vi "Host_HealthCheck_convertCluster.vi"(11 "Data":T1={"cRIO Data"={"HallEffect Right (cm)"=0.0, "HallEffect Left (cm)"=0.0, "Optical Sensor 1 (V)"=0.0, "Optical Sensor 2 (V)"=0.0, "24V Voltage  (V)"=0.0, "24V Current (A)"=0.0, "Contactor H1 Continuity"=0.0, "Contactor L1 Continuity "=0.0, "Contactor H2 Continuity"=0.0, "Contactor L2 Continuity "=0.0, "Brake PT(psig)"=0.0, "Pump PT (psig)"=0.0, "24V Temp   (C)"=0.0, "Tank PT(psig) "=0.0, "ABS Pressure 1 (psig)"=0.0, "ABS Pressure 2 (psig) "=0.0, "Displacement (ft)"=0.0, "Velocity (ft/s)"=0.0, "Time (ms)"=0.0, "PV 1 Temp"=0.0, "PV2 Temp"=0.0}, "IMU Data"={"y acceleration (g)"=0.0, "Pressure (psia)"=0.0, "Temperature (F)"=0.0}, "BMS Data"={"Pack 1 Max Cell\n Voltage (V)"=0.0, "Pack 1 Max Cell\n ID "=0.0, "Pack 1 Min Cell \nVoltage (V)"=0.0, "Pack 1 Min Cell \nID "=0.0, "Pack 1 State of Charge  (%)"=0.0, "Pack 1 Average Voltage1 (V)"=0.0, "Pack 1Voltage Delta (V)"=0.0, "Pack 1 Current (A)"=0.0, "Pack 1 Voltage (V)"=0.0, "Pack 1 Max Resistance (Ohm)"=0.0, "Pack 1Min Resistance (Ohm)"=0.0, "Pack 1Average Resistance (Ohm)"=0.0, "Pack 1Delta Resistance (Ohm)"=0.0, "Pack 1 Highest Temperature(F)"=0.0, "BmsStatus1"={"isFault"=FALSE, "isolationMonitoring"=FALSE}, "Pack 2 Max Cell\n Voltage (V) "=0.0, "Pack 2 Max Cell\n ID  "=0.0, "Pack 2 Min Cell \nVoltage (V) "=0.0, "Pack 2 Min Cell \nID  "=0.0, "Pack 2 Average Voltage1 (V)"=0.0, "Pack 2 Voltage Delta (V) "=0.0, "Pack 2 Current (A)"=0.0, "Pack 2 Voltage (V) "=0.0, "Pack 2 State of Charge  (%) "=0.0, "Pack 2 Max Resistance (Ohm) "=0.0, "Pack 2 Min Resistance (Ohm)"=0.0, "Pack 2 Average Resistance (Ohm)"=0.0, "Pack 2 Delta Resistance (Ohm) "=0.0, "Pack 2 Highest Temperature(F) "=0.0, "BmsStatus 2"={"isFault"=FALSE, "isolationMonitoring"=FALSE}}, "Motor Data"={" Velocity (RPM)"=0.0, " MotorTemp(C)"=0.0, " ControlTemp(C)"=0.0, " DcLinkVolt(V)"=0.0, " ErrorCode"=0.0, "IsAlive"=FALSE, "motorStatus"={"isReady"=FALSE, "isOn"=FALSE, "isOperEn"=FALSE, "isFault"=FALSE, "isVoltEn"=FALSE, "targetReached"=FALSE, "isWarning"=FALSE}, "motorControllerState"=1}} {"Motor Data"."motorControllerState" items=["unknown"=1, "boot-up"=0, "stopped"=4, "operational"=5, "pre-operational"=127, "connection lost"=128]}) -> (3 "Array":dbl[](array[numeric]))   [LabVIEW 2018]
uses:
  Type_Def/TypeDef_cRIODatas.ctl
  Type_Def/TypeDef_BMSDatas.ctl
  Type_Def/Master_DataControl.ctl
  Type_Def/TypeDef FixedMotorData.ctl
  Type_Def/Type_Def IMUDatas.ctl
  Type_Def/TypeDef_BMSStatuss.ctl
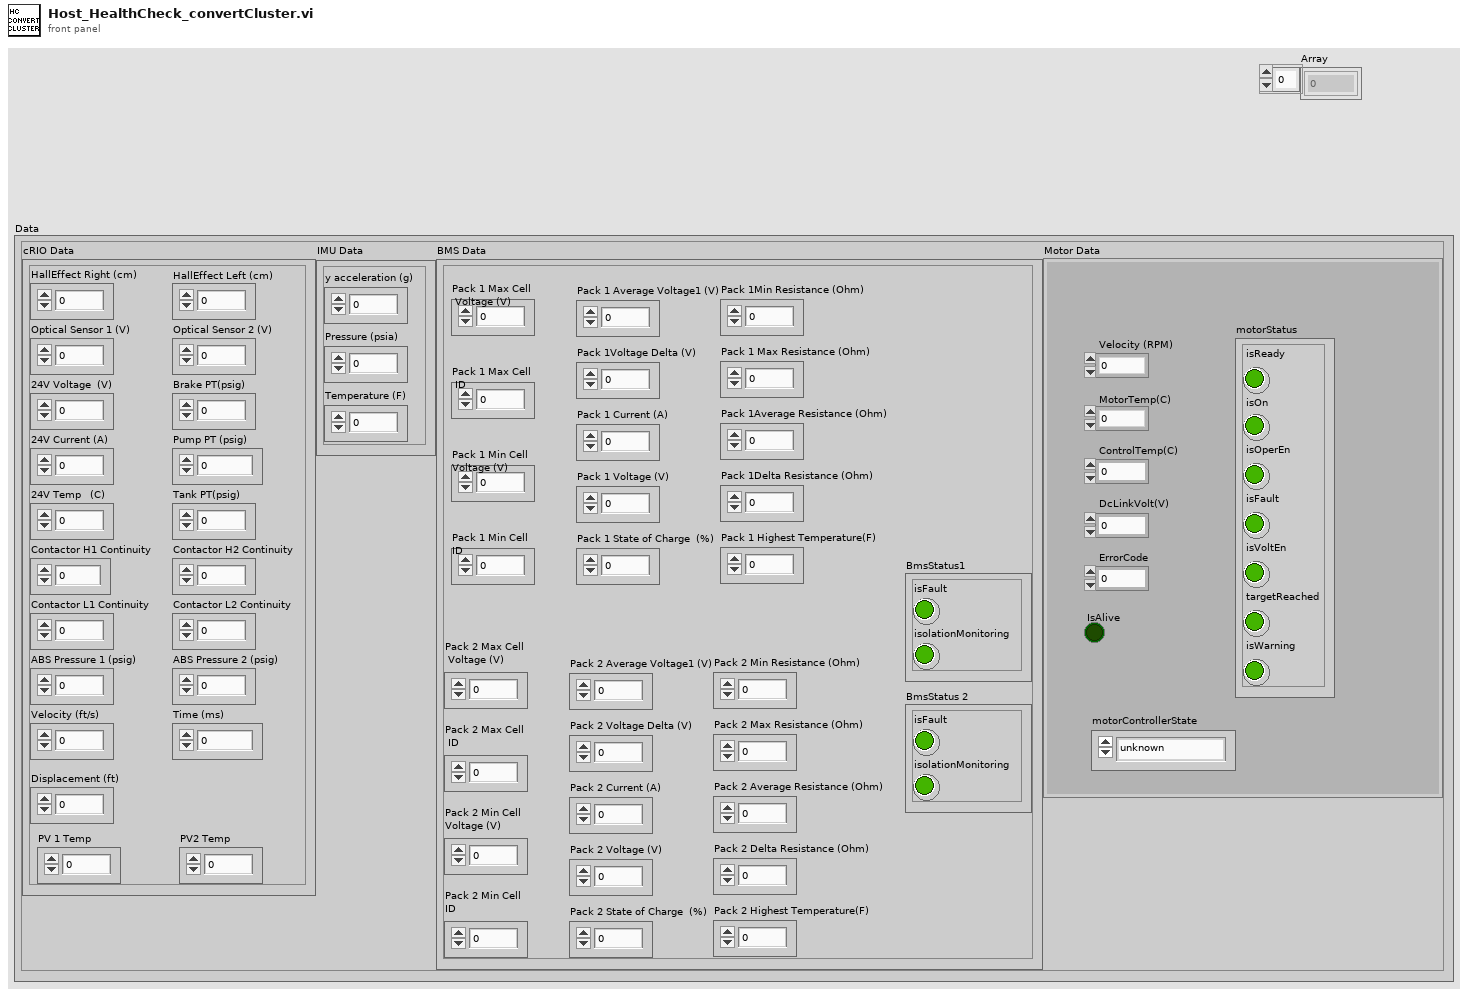
[diagram p1: front panel]
types:
  T1 = typedef "Master_DataControl.ctl" = cluster{"cRIO Data":T2, "IMU Data":T3, "BMS Data":T4, "Motor Data":T6}
  T2 = typedef "TypeDef_cRIODatas.ctl" = cluster{"HallEffect Right (cm)":dbl, "HallEffect Left (cm)":dbl, "Optical Sensor 1 (V)":dbl, "Optical Sensor 2 (V)":dbl, "24V Voltage  (V)":dbl, "24V Current (A)":dbl, "Contactor H1 Continuity":dbl, "Contactor L1 Continuity ":dbl, "Contactor H2 Continuity":dbl, "Contactor L2 Continuity ":dbl, "Brake PT(psig)":dbl, "Pump PT (psig)":dbl, "24V Temp   (C)":dbl, "Tank PT(psig) ":dbl, "ABS Pressure 1 (psig)":dbl, "ABS Pressure 2 (psig) ":dbl, "Displacement (ft)":dbl, "Velocity (ft/s)":dbl, "Time (ms)":dbl, "PV 1 Temp":dbl, "PV2 Temp":dbl}
  T3 = typedef "Type_Def IMUDatas.ctl" = cluster{"y acceleration (g)":dbl, "Pressure (psia)":dbl, "Temperature (F)":dbl}
  T4 = typedef "TypeDef_BMSDatas.ctl" = cluster{"Pack 1 Max Cell\n Voltage (V)":dbl, "Pack 1 Max Cell\n ID ":dbl, "Pack 1 Min Cell \nVoltage (V)":dbl, "Pack 1 Min Cell \nID ":dbl, "Pack 1 State of Charge  (%)":dbl, "Pack 1 Average Voltage1 (V)":dbl, "Pack 1Voltage Delta (V)":dbl, "Pack 1 Current (A)":dbl, "Pack 1 Voltage (V)":dbl, "Pack 1 Max Resistance (Ohm)":dbl, "Pack 1Min Resistance (Ohm)":dbl, "Pack 1Average Resistance (Ohm)":dbl, "Pack 1Delta Resistance (Ohm)":dbl, "Pack 1 Highest Temperature(F)":dbl, "BmsStatus1":T5, "Pack 2 Max Cell\n Voltage (V) ":dbl, "Pack 2 Max Cell\n ID  ":dbl, "Pack 2 Min Cell \nVoltage (V) ":dbl, "Pack 2 Min Cell \nID  ":dbl, "Pack 2 Average Voltage1 (V)":dbl, "Pack 2 Voltage Delta (V) ":dbl, "Pack 2 Current (A)":dbl, "Pack 2 Voltage (V) ":dbl, "Pack 2 State of Charge  (%) ":dbl, "Pack 2 Max Resistance (Ohm) ":dbl, "Pack 2 Min Resistance (Ohm)":dbl, "Pack 2 Average Resistance (Ohm)":dbl, "Pack 2 Delta Resistance (Ohm) ":dbl, "Pack 2 Highest Temperature(F) ":dbl, "BmsStatus 2":T5}
  T5 = typedef "TypeDef_BMSStatuss.ctl" = cluster{"isFault":bool, "isolationMonitoring":bool}
  T6 = typedef "TypeDef FixedMotorData.ctl" = cluster{" Velocity (RPM)":dbl, " MotorTemp(C)":dbl, " ControlTemp(C)":dbl, " DcLinkVolt(V)":dbl, " ErrorCode":dbl, "IsAlive":bool, "motorStatus":cluster{"isReady":bool, "isOn":bool, "isOperEn":bool, "isFault":bool, "isVoltEn":bool, "targetReached":bool, "isWarning":bool}, "motorControllerState":u16}
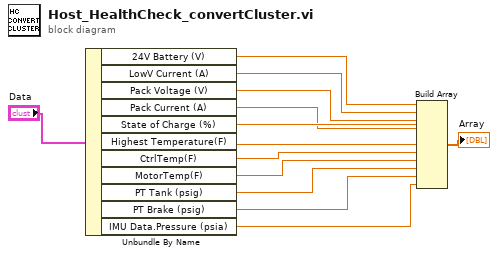
[diagram p0: block diagram]
diagram:
  n1 = Unbundle By Name("Data") -> ("24V Battery (V)"=w4:dbl, "LowV Current (A)"=w5:dbl, "Pack Voltage (V)"=w6:dbl, "Pack Current (A)"=w9:dbl, "State of Charge (%)"=w10:dbl, "Highest Temperature(F)"=w11:dbl, "CtrlTemp(F)"=w12:dbl, "MotorTemp(F)"=w8:dbl, "PT Tank (psig)"=w3:dbl, "PT Brake (psig)"=w2:dbl, "IMU Data.Pressure (psia)"=w1:dbl)
  n2 = Build Array(w4, w5, w6, w9, w10, w11, w12, w8, w3, w2, w1) -> (→"Array":dbl[])
